vi "Create Observer.vi"(8 "Additional Input":refnum<class "Send.lvclass">, 9 "Input":refnum<class "Send.lvclass">) -> (3 "Observer":refnum<class "Observer.lvclass">)   [LabVIEW 2011, in "Messenging.lvlib" / "ObserverSet.lvclass"]
uses:
  ObserverSet.lvclass
  Send/Send.lvclass
  SendOnly/Observer.lvclass
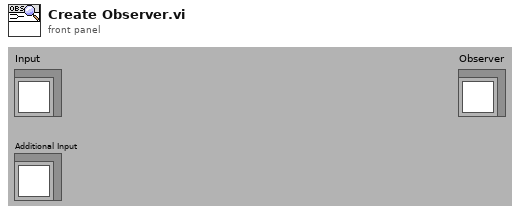
[diagram p1: front panel]
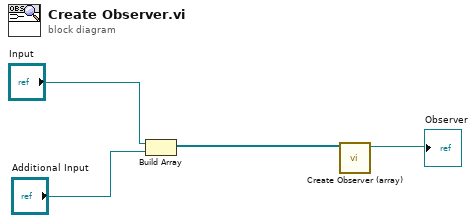
[diagram p0: block diagram]
diagram:
  n1 = Build Array("Input", "Additional Input") -> (w2:refnum<class "Send.lvclass">[])
  n2 = call "Create Observer (array).vi"("Array of Input"=w2) -> ("Observer"=→"Observer":refnum<class "Observer.lvclass">)  [unwired: 2 in, 6 out]
